vi "BK Precision SCPI 169XB Output DC Volts.vi"() -> ()   [LabVIEW 2021]
doc: "This example shows how to configure the instrument's output voltage level, over current protection, and over voltage protection. The actual voltage level and actual current level are returned as well as whether over voltage protection (OVP) or over current protection (OCP) has been tripped."
uses:
  BK Precision 169XB.lvlib
panel:
  out "Meas Power (P)":dbl format="%.3g"
  in  "Serial Configuration":T1={"Baud Rate"=9600, "Parity"=0, "Data Bits"=8, "Stop Bits"=10, "Flow Control"=0} {"Flow Control" items=["None", "XON/XOFF", "RTS/CTS", "XON/XOFF & RTS/CTS", "DTR/DSR", "XON/XOFF & DTR/DSR"]; "Stop Bits" items=["1.0"=10, "1.5"=15, "2.0"=20]; "Data Bits" items=["7"=7, "8"=8]; "Parity" items=["None", "Odd", "Even", "Mark", "Space"]; "Baud Rate" items=["300"=300, "600"=600, "1200"=1200, "2400"=2400, "4800"=4800, "9600"=9600, "19200"=19200]}
  in  "Set Voltage":dbl format="%.1g"
  in  "Set Current":dbl format="%.1g"
  in  "SOVP":dbl format="%0.1f"
  in  "Stop Output":bool
  out "Meas Current Limit (A)":dbl format="%.2f"
  out "Meas Voltage Level (V)":dbl format="%.2f"
  in  "VISA resource name":refnum<visa-resource-name>
  # "(c) 2014 <Enter Company Name Here>.  ALL RIGHTS RESERVED."
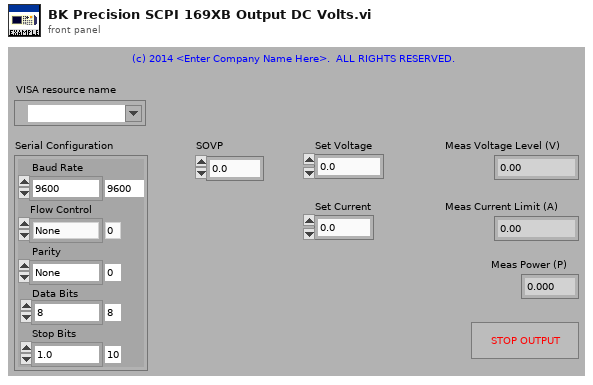
[diagram p1: front panel]
types:
  T1 = cluster{"Baud Rate":u32, "Parity":u16, "Data Bits":u16, "Stop Bits":u16, "Flow Control":u16}
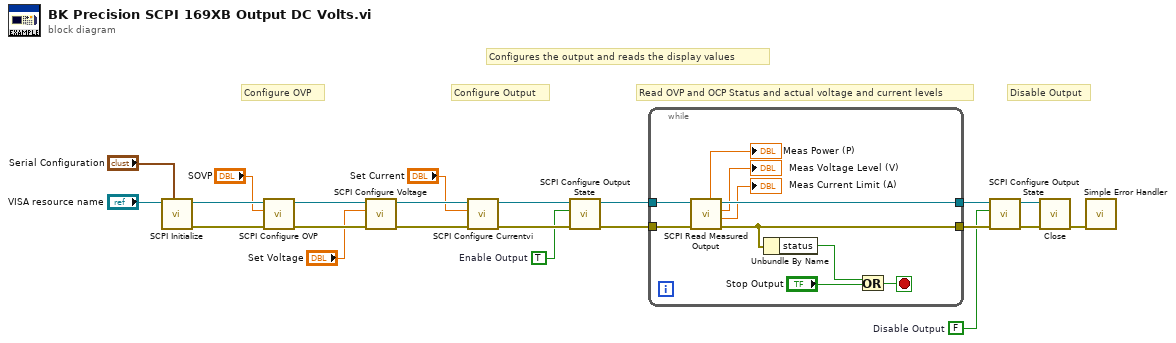
[diagram p0: block diagram]
diagram:
  w1 = FALSE  # Disable Output
  w11 = TRUE  # Enable Output
  # "Configures the output and reads the display values"
  # "Disable Output"
  # "Read OVP and OCP Status and actual voltage and current levels"
  # "Configure Output"
  # "Configure OVP"
  n1 = call "SCPI Initialize.vi"("Serial Configuration"="Serial Configuration", "VISA resource name"="VISA resource name") -> ("error out"=w16:errorcluster, "VISA resource name out"=w15:refnum<visa-resource-name>)  [unwired: 8 in]
  n2 = call "SCPI Configure OVP.vi"("error in (no error)"=w16, "Set Current"="SOVP", "VISA resource name"=w15) -> ("error out"=w17:errorcluster, "VISA resource name out"=w14:refnum<visa-resource-name>)  [unwired: 7 in]
  n3 = call "SCPI Configure Voltage.vi"("error in (no error)"=w17, "Set Voltage"="Set Voltage", "VISA resource name"=w14) -> ("error out"=w18:errorcluster, "VISA resource name out"=w13:refnum<visa-resource-name>)  [unwired: 7 in]
  n4 = call "SCPI Configure Currentvi.vi"("error in (no error)"=w18, "Set Current"="Set Current", "VISA resource name"=w13) -> ("error out"=w19:errorcluster, "VISA resource name out"=w12:refnum<visa-resource-name>)  [unwired: 7 in]
  n5 = call "SCPI Configure Output State.vi"("error in (no error)"=w19, "Enable Output (T: Enable)"=w11, "VISA resource name"=w12) -> ("error out"=w20:errorcluster, "VISA resource name out"=w6:refnum<visa-resource-name>)  [unwired: 7 in]
  n6 = while {
    tunnel: [w29] -> w4
    tunnel: [w26] -> w5
    tunnel: w20 -> [w24]
    tunnel: w6 -> [w25]
    stop <- w32 stop-if-true
    n7 = call "SCPI Read Measured Output.vi"("error in (no error)"=w24, "VISA resource name"=w25) -> ("error out"=w26:errorcluster, "Meas Current"=→"Meas Current Limit (A)":dbl, "Meas Voltage"=→"Meas Voltage Level (V)":dbl, "VISA resource name out"=w29:refnum<visa-resource-name>, "Meas Power"=→"Meas Power (P)":dbl)  [unwired: 5 in]
    n8 = Unbundle By Name(w26) -> ("status"=w30:bool)
    n9 = Or(x=w30, y="Stop Output") -> (x .or. y?=w32:bool)
  }
  n10 = call "SCPI Configure Output State.vi"("error in (no error)"=w5, "Enable Output (T: Enable)"=w1, "VISA resource name"=w4) -> ("error out"=w2:errorcluster, "VISA resource name out"=w3:refnum<visa-resource-name>)  [unwired: 7 in]
  n11 = call "Close.vi"("error in (no error)"=w2, "VISA resource name"=w3) -> ("error out"=w22:errorcluster)  [unwired: 9 in]
  n12 = call <vilib>:"Simple Error Handler.vi"("error in (no error)"=w22) -> ()  [unwired: 4 in, 5 out]
